vi "f23.vi"() -> ()   [LabVIEW 2014]
panel:
  in  "f23":dbl
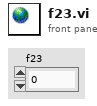
[diagram p1: front panel]
diagram:
